vi "Check Staff.vi"(0 "File Data Manager in":refnum<class "File Data Manager.lvclass">, 11 "error in (no error)":errorcluster) -> (4 "File Data Manager out":refnum<class "File Data Manager.lvclass">, 15 "error out":errorcluster)   [LabVIEW 2023, in "File Data Manager.lvlib" / "File Data Manager.lvclass"]
uses:
  File Data Manager.lvclass
  File Data Manager.lvclass/File Data Manager.ctl
  Central Data Manager/Central Data Manager/Staff Designation.ctl
  Central Data Manager/Central Data Manager/Central Data Manager.lvclass
  <vilib>/ActorFramework/Actor/Actor.lvclass
  Interfaces/Incoming Hotel Management Tool Model Interface Messages/Available Staffs Msg/Available Staffs Msg.lvclass
  C:/Users/bhaghyaraj/Trainings/NI Actor Framework/SDLC/Central Data Manager/Central Data Manager/Central Data Manager.lvclass
  C:/Users/bhaghyaraj/Trainings/NI Actor Framework/SDLC/Model Base/Model Base/Model Base.lvclass
  C:/Program Files/National Instruments/LabVIEW 2023/vi.lib/ActorFramework/Actor/Actor.lvclass
  C:/Users/bhaghyaraj/Trainings/NI Actor Framework/SDLC/Interfaces/Model Base/Incoming Model Base Interface.lvclass
  C:/Users/bhaghyaraj/Trainings/NI Actor Framework/SDLC/File Data Manager/File Data Manager/File Data Manager.lvclass
  Room Service Types/Room Service Base/Room Service Base.lvclass
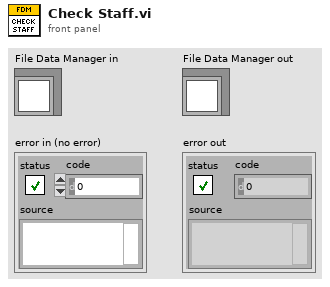
[diagram p1: front panel]
types:
  T1 = typedef "Central Data Manager.lvlib/Central Data Manager.lvclass/Staff Designation.ctl" = enum16{"Manager", "Receptionist", "Chef", "Waiter", "Room Service"}
  T2 = typedef "Central Data Manager.lvlib/Central Data Manager.lvclass/Staff Details.ctl" = cluster{"Staff Name":string, "Designation":T1, "Attendance":T3}
  T3 = typedef "Central Data Manager.lvlib/Central Data Manager.lvclass/Staff Attendance.ctl" = enum16{"Present", "Absent"}
  T4 = map{string, map{string, refnum<class "Room Service Base.lvclass">}}
  T5 = map{string, refnum<class "Room Service Base.lvclass">}
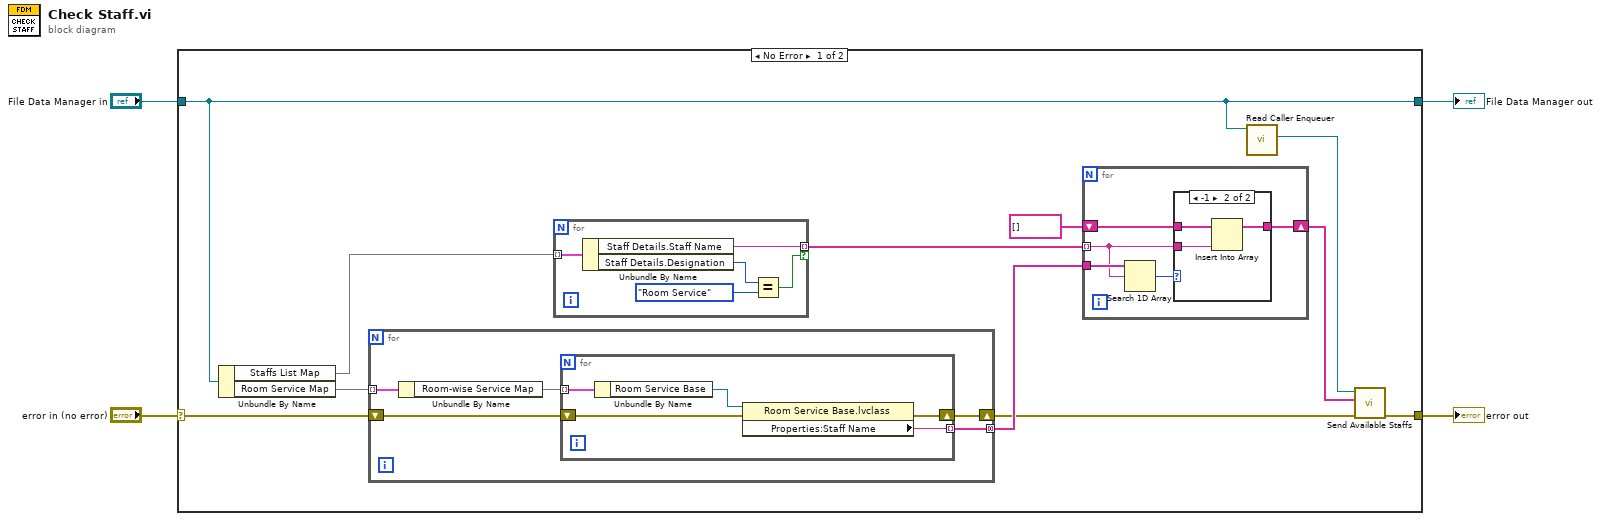
[diagram p0: block diagram]
diagram:
  n1 = case shown="No Error" "error in (no error)" {
    selector: "error in (no error)" -> [w13 w40]
    tunnel: "File Data Manager in" -> [w9 w41]
    tunnel: [w9 w41] -> w2
    tunnel: [w7 w40] -> w1
    frame No Error {
      n2 = Unbundle By Name(w9) -> ("Staffs List Map"=w14:map{string, T2}, "Room Service Map"=w15:T4)
      n3 = for {
        tunnel: w15 -> [w34] mode=indexing
        shift-right: [w31] -> w8
        shift-left: w13 -> [w32]
        tunnel: [w30] -> w10 mode=concatenating
        n4 = Unbundle By Name(w34) -> ("Room-wise Service Map"=w33:T5)
        n5 = for {
          tunnel: w33 -> [w39] mode=indexing
          shift-right: [w36] -> w31
          shift-left: w32 -> [w37]
          tunnel: [w35] -> w30 mode=indexing
          n6 = Unbundle By Name(w39) -> ("Room Service Base"=w38:refnum<class "Room Service Base.lvclass">)
          n7 = property class="Room Service Base.lvclass"(reference=w38, error in=w37) -> (error out=w36:errorcluster, "Properties:Staff Name"=w35:string)  [unwired: 1 out]
        }
      }
      n8 = for {
        tunnel: w14 -> [w29] mode=indexing
        tunnel: [w28] -> w12 mode=indexing if=w27
        n9 = Unbundle By Name(w29) -> ("Staff Details.Staff Name"=w28:string, "Staff Details.Designation"=w26:T1)
        n10 = Equal?(x=w26, y=Staff_Designation."Room Service") -> (x = y?=w27:bool)
      }
      n11 = for {
        tunnel: w12 -> [w17] mode=indexing
        shift-right: [w19] -> w5
        shift-left: string[] [] -> [w20]
        tunnel: w10 -> [w18]
        n12 = Search 1D Array(1D array=w18, element=w17) -> (index of element=w16:i32)  [unwired: 1 in]
        n13 = case shown="-1" w16 {
          tunnel: w20 -> [w21 w24]
          tunnel: [w21 w23] -> w19
          tunnel: w17 -> [_ w22]
          frame Default {
          }
          frame -1 {
            n14 = Insert Into Array(array=w24, new element=w22) -> (w23:string[])  [unwired: 1 in]
          }
        }
      }
      n15 = call <vilib>:"Read Caller Enqueuer.vi"("Actor"=w9) -> ("Caller Enqueuer"=w6:refnum<class "Message Enqueuer.lvclass">)  [unwired: 10 in]
      n16 = call "Send Available Staffs.vi"("error in (no error)"=w8, "Staff Name"=w5, "Message Enqueuer"=w6) -> ("error out"=w7:errorcluster)  [unwired: 7 in, 1 out]
    }
    frame Error {
    }
  }
  "error out" <- w1
  "File Data Manager out" <- w2
